vi "CTRE_Phoenix_MotorControl_PushMotionProfileTrajectory_3.vi"(8 "error in":errorcluster, 10 "Trajectory Point":T1, 11 "PhoenixMotorControlDevRef":T2={"DeviceStatus"={"status"=FALSE, "code"=0, "source"=""}, "Type"=enum."PWM", "PWM"={"PWM Channel"=enum."Invalid", "DeadBand"={"Name"="", "maxPositivePwm"=0, "minPositivePwm"=0, "centerPwm"=0, "maxNegativePwm"=0, "minNegativePwm"=0, "angularRange"=0}}, "CAN"={"Device Number"=0, "SetOutput VI Ref"=variant(enum8{"Percent VBus", "Current", "Speed", "Position", "Voltage"} enum."Percent VBus"), "GetOutput VI Ref"=variant(refnum<k1> refnum), "Enable VI Ref"=variant(dbl 12.0), "Disable VI Ref"=variant(enum8{"Percent VBus", "Speed", "Position", "Slave", "Unchanged / Invalid", "Voltage Compensation", "Current", "Motion Profile"} enum."Percent VBus"), "Data"=variant}, "Invert"=FALSE, "DIO PWM"={"PWM \"Enable\" Channel"=enum."Invalid", "DIOChannel"=enum."Invalid", "PWM Rate"=0.0}}) -> (0 "error out":errorcluster, 3 "PhoenixMotorControlDevRef":T2={"DeviceStatus"={"status"=FALSE, "code"=0, "source"=""}, "Type"=enum."PWM", "PWM"={"PWM Channel"=enum."Invalid", "DeadBand"={"Name"="", "maxPositivePwm"=0, "minPositivePwm"=0, "centerPwm"=0, "maxNegativePwm"=0, "minNegativePwm"=0, "angularRange"=0}}, "CAN"={"Device Number"=0, "SetOutput VI Ref"=variant(enum8{"Percent VBus", "Current", "Speed", "Position", "Voltage"} enum."Percent VBus"), "GetOutput VI Ref"=variant(refnum<k1> refnum), "Enable VI Ref"=variant(dbl 12.0), "Disable VI Ref"=variant(enum8{"Percent VBus", "Speed", "Position", "Slave", "Unchanged / Invalid", "Voltage Compensation", "Current", "Motion Profile"} enum."Percent VBus"), "Data"=variant}, "Invert"=FALSE, "DIO PWM"={"PWM \"Enable\" Channel"=enum."Invalid", "DIOChannel"=enum."Invalid", "PWM Rate"=0.0}})   [LabVIEW 2020]
doc: "Push another trajectory point into the top level buffer (which is emptied\ninto the motor controller's bottom buffer as room allows).\n\nThe members should be filled in with these values...\n\n <b>position</b> servo position in sensor units.\n <b>velocity</b> velocity to feed-forward in sensor units per 100ms.\n <b>arbFeedFwd</b> Arbitrary Feed-forward (from -1 to 1) for the primary PID loop.\n <b>auxPosition</b> servo position in sensor units for the auxiliary PID loop.\n <b>auxVelocity</b> velocity to feed-forward in sensor units per 100ms.\n <b>auxArbFeedFwd</b> arbitrary feed-forward (from -1 to 1) for the auxiliary PID loop.\n <b>profileSlotSelect0</b> Which slot to get PIDF gains.\n PID is used for position servo.\n F is used as the Kv constant for velocity feed-forward.\n Typically this is hardcoded to the a particular slot, but you are free\n gain schedule if need be.\n Choose from [0,3].\n <b>profileSlotSelect1</b> Which slot to get PIDF gains for auxiliary PID.\n This only has impact during MotionProfileArc Control mode.\n Choose from [0,1].\n <b>isLastPoint</b> Set to true to signal Talon that this is the final point, so do not\n attempt to pop another trajectory point from out of the Talon buffer.\n Instead continue processing this way point. Typically the velocity\n member variable should be zero so that the motor doesn't spin indefinitely.\n <b>zeroPos</b> set to nonzero to signal motor controller to \"zero\" the selected\n position sensor before executing this trajectory point.\n Typically the first point should have this set only thus\n allowing the remainder of the MP positions to be relative to\n zero.\n <b>durationMs</b> Duration to apply this trajectory pt.\n This time unit is ADDED to the exising base time set by\n the ConfigMotionProfileTrajectoryPeriod VI.\n <b>useAuxPID?</b> must be set to TRUE to use auxiliary PID for motion profiling.\n Should be set to FALSE if using traditional motion profile."
uses:
  <vilib>/Rock Robotics/WPI/MotorControl/WPI_MotorControlDeviceRef.ctl
  <vilib>/Rock Robotics/WPI/MotorControl/WPI_MotorControlType.ctl
  <vilib>/Rock Robotics/SystemInterfaces/DIO/FPGA_DIOPWMChannel.ctl
  <vilib>/Rock Robotics/WPI/PWM/WPI_PWMDeadband.ctl
  <vilib>/Rock Robotics/SystemInterfaces/DIO/FPGA_DIOChannel.ctl
  <vilib>/Rock Robotics/WPI/ThirdParty/Phoenix-LabVIEW/Motor Controller/Controls/CTRE_Phoenix_MotorControl_MotionProfileTrajectoryPoint.ctl
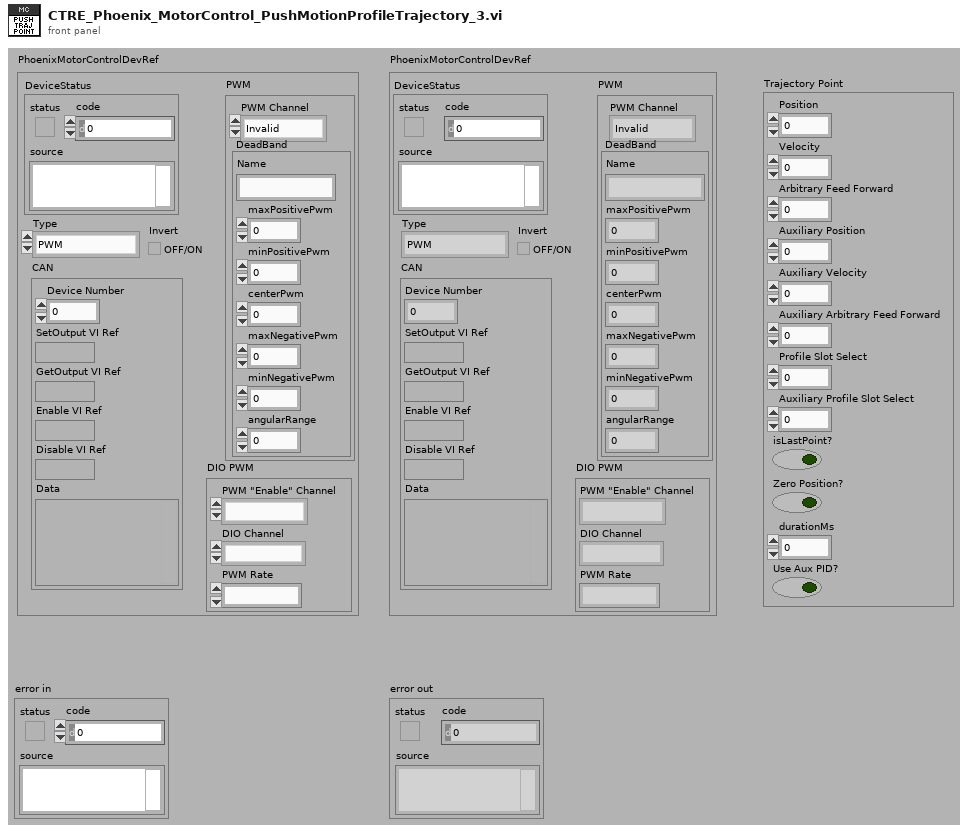
[diagram p1: front panel]
types:
  T1 = typedef "CTRE_Phoenix_MotorControl_MotionProfileTrajectoryPoint.ctl" = cluster{"Position":dbl, "Velocity":dbl, "Arbitrary Feed Forward":dbl, "Auxiliary Position":dbl, "Auxiliary Velocity":dbl, "Auxiliary Arbitrary Feed Forward":dbl, "Profile Slot Select":i32, "Auxiliary Profile Slot Select":i32, "isLastPoint?":bool, "Zero Position?":bool, "durationMs":u32, "Use Aux PID?":bool}
  T2 = typedef "WPI_MotorControlDeviceRef.ctl" = cluster{"DeviceStatus":errorcluster, "Type":T3, "PWM":cluster{"PWM Channel":T4, "DeadBand":T5}, "CAN":cluster{"Device Number":u8, "SetOutput VI Ref":variant, "GetOutput VI Ref":variant, "Enable VI Ref":variant, "Disable VI Ref":variant, "Data":variant}, "Invert":bool, "DIO PWM":cluster{"PWM \"Enable\" Channel":T4, "DIOChannel":T6, "PWM Rate":dbl}}
  T3 = typedef "WPI_MotorControlType.ctl" = enum16{"PWM", "CAN", "DIO PWM"}
  T4 = typedef "FPGA_DIOPWMChannel.ctl" = enum8{"PWM 0", "PWM 1", "PWM 2", "PWM 3", "PWM 4", "PWM 5", "PWM 6", "PWM 7", "PWM 8", "PWM 9", "PWM MXP 0", "PWM MXP 1", "PWM MXP 2", "PWM MXP 3", "PWM MXP 4", "PWM MXP 5", "PWM MXP 6", "PWM MXP 7", "PWM MXP 8", "PWM MXP 9", "Invalid"}
  T5 = typedef "WPI_PWMDeadband.ctl" = cluster{"Name":string, "maxPositivePwm":i32, "minPositivePwm":i32, "centerPwm":i32, "maxNegativePwm":i32, "minNegativePwm":i32, "angularRange":u16}
  T6 = typedef "FPGA_DIOChannel.ctl" = enum8{"DIO 0", "DIO 1", "DIO 2", "DIO 3", "DIO 4", "DIO 5", "DIO 6", "DIO 7", "DIO 8", "DIO 9", "DIO MXP 0", "DIO MXP 1", "DIO MXP 2", "DIO MXP 3", "DIO MXP 4", "DIO MXP 5", "DIO MXP 6", "DIO MXP 7", "DIO MXP 8", "DIO MXP 9", "DIO MXP 10", "DIO MXP 11", "DIO MXP 12", "DIO MXP 13", "DIO MXP 14", "DIO MXP 15", "SPI Port CS1", "SPI Port CS2", "SPI Port CS3", "SPI Port MISO", "SPI Port MOSI", "Invalid"}
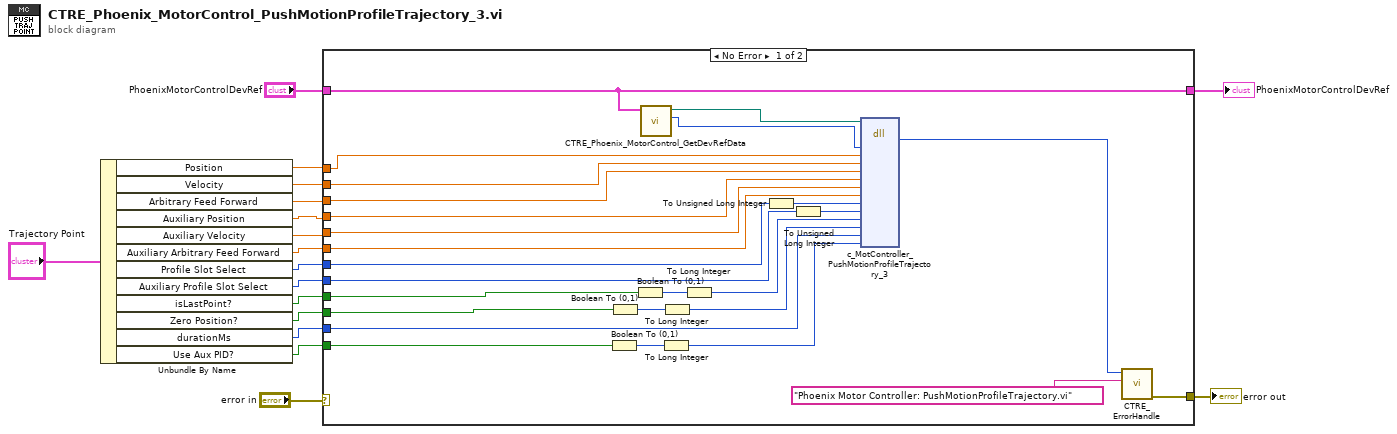
[diagram p0: block diagram]
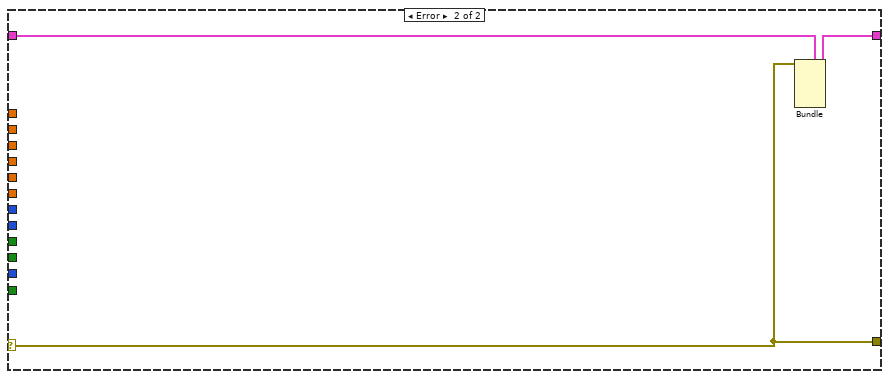
[diagram p2: hidden frame]
diagram:
  n1 = Unbundle By Name("Trajectory Point") -> ("Position"=w12:dbl, "Velocity"=w11:dbl, "Arbitrary Feed Forward"=w10:dbl, "Auxiliary Position"=w9:dbl, "Auxiliary Velocity"=w8:dbl, "Auxiliary Arbitrary Feed Forward"=w7:dbl, "Profile Slot Select"=w6:i32, "Auxiliary Profile Slot Select"=w5:i32, "isLastPoint?"=w4:bool, "Zero Position?"=w3:bool, "durationMs"=w2:u32, "Use Aux PID?"=w1:bool)
  n2 = case shown="No Error" "error in" {
    selector: "error in" -> [_ w45]
    tunnel: "PhoenixMotorControlDevRef" -> [w43 w46]
    tunnel: [w41 w45] -> w16
    tunnel: [w43 w44] -> w14
    tunnel: w6 -> [w27 _]
    tunnel: w4 -> [w38 _]
    tunnel: w3 -> [w36 _]
    tunnel: w12 -> [w33 _]
    tunnel: w11 -> [w32 _]
    tunnel: w9 -> [w31 _]
    tunnel: w5 -> [w26 _]
    tunnel: w2 -> [w21 _]
    tunnel: w10 -> [w30 _]
    tunnel: w8 -> [w29 _]
    tunnel: w7 -> [w28 _]
    tunnel: w1 -> [w19 _]
    frame No Error {
      n3 = Boolean To (0,1)(Boolean=w19) -> (0, 1=w20:i16)
      n4 = Boolean To (0,1)(Boolean=w36) -> (0, 1=w35:i16)
      n5 = Boolean To (0,1)(Boolean=w38) -> (0, 1=w37:i16)
      n6 = call <vilib>:"CTRE_Phoenix_MotorControl_GetDevRefData.vi"("PhoenixMotorControlDevRef"=w43) -> ("handle"=w34:u64, "Library"=w42:path)  [unwired: 4 in, 5 out]
      n7 = To Long Integer(number=w20) -> (32bit integer=w18:i32)
      n8 = To Long Integer(number=w35) -> (32bit integer=w22:i32)
      n9 = To Long Integer(number=w37) -> (32bit integer=w23:i32)
      n10 = To Unsigned Long Integer(number=w27) -> (unsigned 32bit integer=w25:u32)
      n11 = To Unsigned Long Integer(number=w26) -> (unsigned 32bit integer=w24:u32)
      n12 = dll-call lib="?" fn="c_MotController_PushMotionProfileTrajectory_3"(path in=w42, "handle"=w34, "position"=w33, "velocity"=w32, "arbFeedFwd"=w30, "auxiliaryPos"=w31, "auxiliaryVel"=w29, "auxiliaryArbFeedFwd"=w28, "profileSlotSelect0"=w25, "profileSlotSelect1"=w24, "isLastPoint"=w23, "zeroPos"=w22, "durationMs"=w21, "useAuxPID"=w18) -> ("ErrorCode"=w40:i32)  [unwired: 15 in, 2 out]
      n13 = call <vilib>:"CTRE_ErrorHandle.vi"("origin"="Phoenix Motor Controller: PushMotionProfileTrajectory.vi", "code"=w40) -> ("error out"=w41:errorcluster)  [unwired: 9 in]
    }
    frame Error {
      n14 = Bundle(cluster=w46, "DeviceStatus"=w45) -> (w44:T2)  [unwired: 5 in]
    }
  }
  "PhoenixMotorControlDevRef" <- w14
  "error out" <- w16
